vi "Inlet_Temp_To_Voltage.vi"(0 "Model":enum16{"Estar Centauro", "GFL"}(ring)=enum."GFL", 7 "Temperature":u16=50 max=500, 11 "Error In":errorcluster) -> (6 "Voltage":dbl, 15 "Error Out":errorcluster)   [LabVIEW 2021]
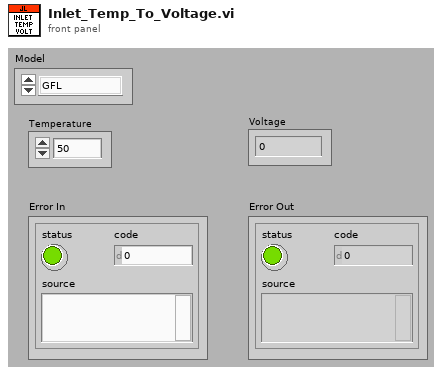
[diagram p1: front panel]
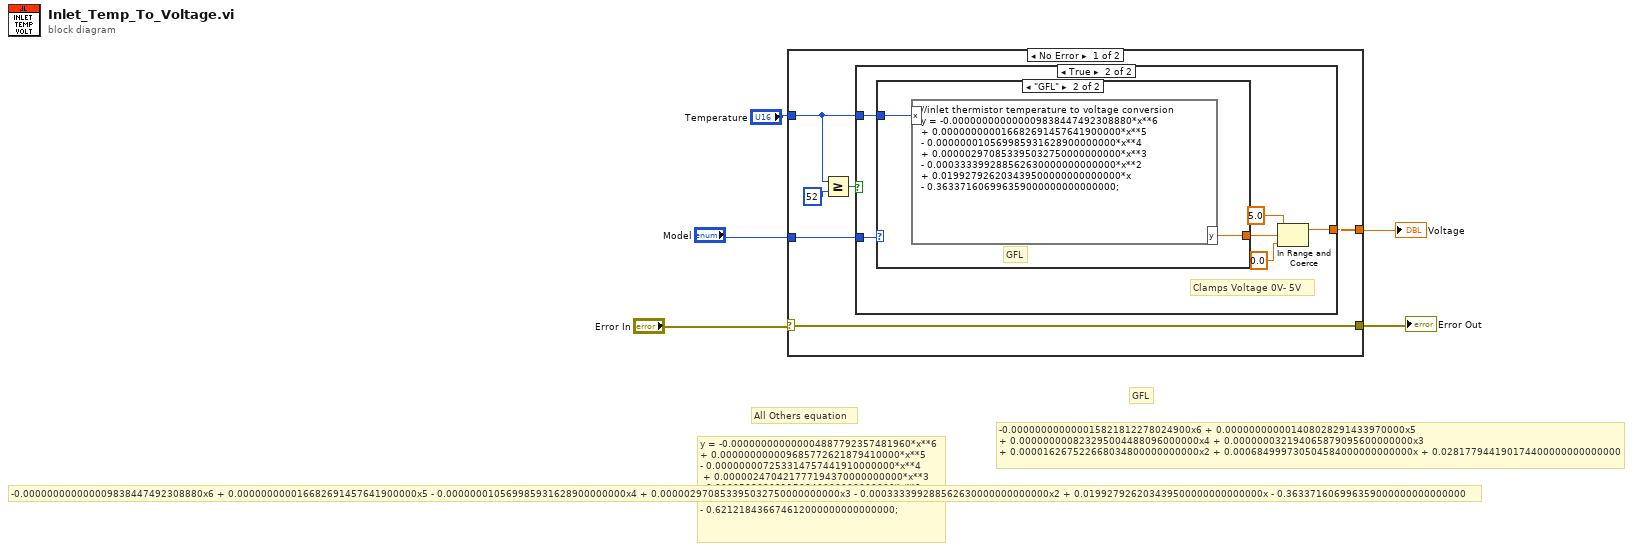
[diagram p0: block diagram]
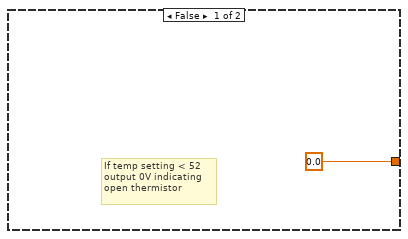
[diagram p2: hidden frame]
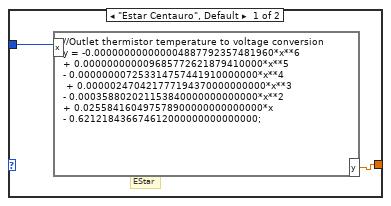
[diagram p3: hidden frame]
diagram:
  # "-0.000000000000009838447492308880x6 + 0.000000000016682691457641900000x5 - 0.000000010569985931628900000000x4 + 0.000002970853395032750000000000x3 - 0.000333399288562630000000000000x2 + 0.019927926203439500000000000000x - 0.363371606996359000000000000000"
  # "-0.000000000000015821812278024900x6 + 0.000000000001408028291433970000x5 \n+ 0.000000000823295004488096000000x4 + 0.000000032194065879095600000000x3 \n+ 0.000016267522668034800000000000x2 + 0.000684999730504584000000000000x + 0.028177944190174400000000000000"
  # "All Others equation"
  # "y = -0.000000000000004887792357481960*x**6 \n+ 0.000000000009685772621879410000*x**5 \n- 0.000000007253314757441910000000*x**4\n + 0.000002470421777194370000000000*x**3 \n- 0.000358802021153840000000000000*x**2 \n+ 0.025584160497578900000000000000*x \n- 0.621218436674612000000000000000;"
  # "GFL"
  n1 = case shown="No Error" "Error In" {
    selector: "Error In" -> [w11 w23]
    tunnel: "Temperature" -> [w8 _]
    tunnel: [w10 _] -> w5
    tunnel: [w11 w23] -> w4
    tunnel: "Model" -> [w6 _]
    frame No Error {
      n2 = Greater Or Equal?(x=w8, y=u16 52) -> (x >= y?=w9:bool)
      n3 = case shown="True" w9 {
        tunnel: w8 -> [_ w18]
        tunnel: [0.0 ("upper limit") w14] -> w10
        tunnel: w6 -> [_ w13]
        frame False {
          # "If temp setting < 52 \noutput 0V indicating \nopen thermistor"
        }
        frame True {
          # "Clamps Voltage 0V- 5V"
          n4 = case shown="\"GFL\"" w13 {
            tunnel: w18 -> [w19 w22]
            tunnel: [w20 w21] -> w17
            frame "Estar Centauro", Default {
              # "EStar"
              n5 = formula code="//Outlet thermistor temperature to voltage conversion\ny = -0.000000000000004887792357481960*x**6 \n+ 0.000000000009685772621879410000*x**5 \n- 0.000000007253314757441910000000*x**4\n + 0.000002470421777194370000000000*x**3 \n- 0.000358802021153840000000000000*x**2 \n+ 0.025584160497578900000000000000*x \n- 0.621218436674612000000000000000;"("x"=w19) -> ("y"=w20:dbl)
            }
            frame "GFL" {
              # "GFL"
              n6 = formula code="//inlet thermistor temperature to voltage conversion\ny = -0.000000000000009838447492308880*x**6 \n+ 0.000000000016682691457641900000*x**5 \n- 0.000000010569985931628900000000*x**4\n+ 0.000002970853395032750000000000*x**3 \n- 0.000333399288562630000000000000*x**2 \n+ 0.019927926203439500000000000000*x \n- 0.363371606996359000000000000000;"("x"=w22) -> ("y"=w21:dbl)
            }
          }
          n7 = In Range and Coerce(upper limit=5.0, x=w17, lower limit=0.0) -> (coerced(x)=w14:dbl)  [unwired: 1 out]
        }
      }
    }
    frame Error {
    }
  }
  "Voltage" <- w5
  "Error Out" <- w4
